vi "tm_stopcapture.vi"(8 "error in (no error)":errorcluster {"code" format="%.0x"}, 11 "Handle in":u32) -> (0 "error out":errorcluster {"code" format="%.0x"}, 3 "Handle out":u32)   [LabVIEW 2011]
uses:
  tmcamcon.dll
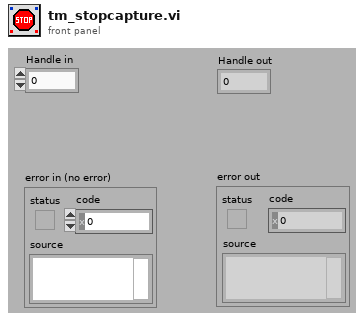
[diagram p1: front panel]
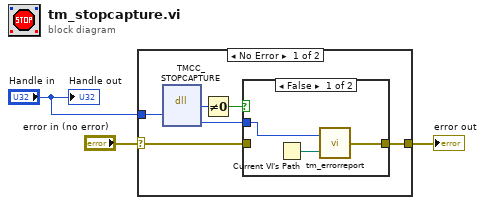
[diagram p0: block diagram]
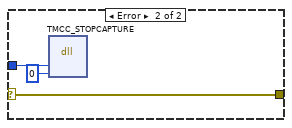
[diagram p3: hidden frame]
diagram:
  n1 = case shown="No Error" "error in (no error)" {
    selector: "error in (no error)" -> [w6 w16]
    tunnel: [w7 w16] -> w2
    tunnel: "Handle in" -> [w8 w14]
    frame No Error {
      n2 = dll-call lib="tmcamcon.dll" fn="TMCC_STOPCAPTURE"("index"=w8) -> ("return type"=w9:u32, "Erval"=w5:i32)  [unwired: 5 in, 2 out]
      n3 = Not Equal To 0?(x=w9) -> (x != 0?=w4:bool)
      n4 = case shown="False" w4 {
        tunnel: w6 -> [_ w13]
        tunnel: [w11 w13] -> w7
        tunnel: w5 -> [w10 _]
        frame False {
          n5 = Current VI's Path() -> (path=w12:path)
          n6 = call <userlib>:"tm_errorreport.vi"("Source"=w12, "Error"=w10) -> ("error out"=w11:errorcluster)
        }
        frame True {
        }
      }
    }
    frame Error {
      n7 = dll-call lib="tmcamcon.dll" fn="TMCC_STOPCAPTURE"("index"=w14, "Erval"=0) -> ()  [unwired: 6 in, 2 out]
    }
  }
  "error out" <- w2
  "Handle out" <- "Handle in"
